vi "CheckRelayClosing.vi"(1 "Converter State":u8(ring) items=["Idle"=0, "Busy"=1, "Wait4srcON"=2, "Ready"=3, "Forming"=5, "Feeding"=6, "Error"=9, "Wait4srcOFF"=10, "ISRC mode"=11, "VSRC mode"=12], 2 "Vdc DC Link":dbl, 3 "Vdc Battery":dbl) -> (0 "Ok to Close Contactor":bool)   [LabVIEW 2017]
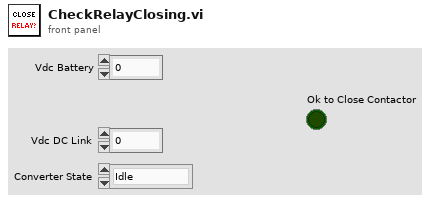
[diagram p1: front panel]
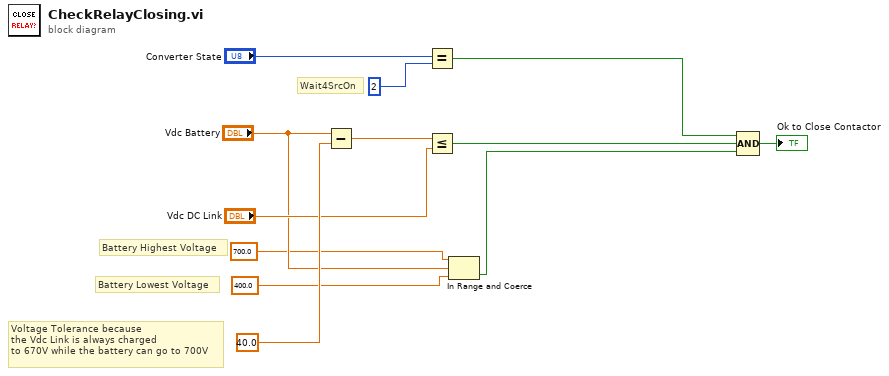
[diagram p0: block diagram]
diagram:
  # "Battery Lowest Voltage"
  # "Battery Highest Voltage"
  # "Wait4SrcOn"
  # "Voltage Tolerance because \nthe Vdc Link is always charged \nto 670V while the battery can go to 700V"
  n1 = Subtract(x="Vdc Battery", y=40.0) -> (x-y=w7:dbl)
  n2 = Equal?(x="Converter State", y=u8 2) -> (x = y?=w10:bool)
  n3 = Less Or Equal?(x=w7, y="Vdc DC Link") -> (x <= y?=w5:bool)
  n4 = In Range and Coerce(upper limit=700.0 ("x"), x="Vdc Battery", lower limit=400.0) -> (In Range?=w1:bool)  [unwired: 1 out]
  n5 = Compound Arithmetic op=AND(w10, w5, w1) -> (→"Ok to Close Contactor":bool)
